vi "Select_UUT_Table.vi"(9 "all Title":string[][](array[string]), 11 "all Table":string[][](array[string])) -> (2 "Title":string[](array[string]), 3 "Table":string[][](array[string]))   [LabVIEW 2017]
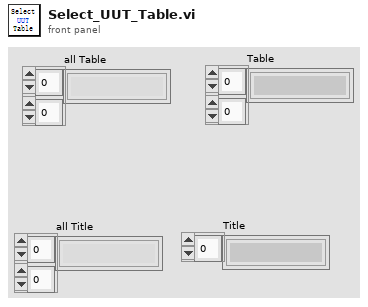
[diagram p1: front panel]
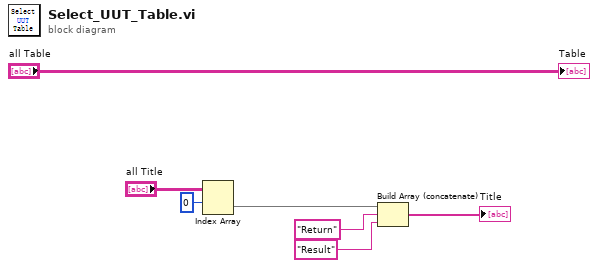
[diagram p0: block diagram]
diagram:
  n1 = Index Array(array="all Title", index (row)=0 ("索引 (行)")) -> (element=w1:string[])  [unwired: 1 in]
  n2 = Build Array (concatenate)(w1, "Return", "Result") -> (→"Title":string[])
  "Table" <- "all Table"
